vi "Set Source Debug Mode.vi"(5 "is Release?":bool=TRUE, 7 "Source Index":i32, 8 "error in (no error)":errorcluster, 11 "ProjectItem in":refnum<vi>) -> (0 "error out":errorcluster, 3 "ProjectItem out":refnum<vi>)   [LabVIEW 2019, in "Project Sync Tools.lvclass"]
uses:
  Project Sync Tools.lvclass
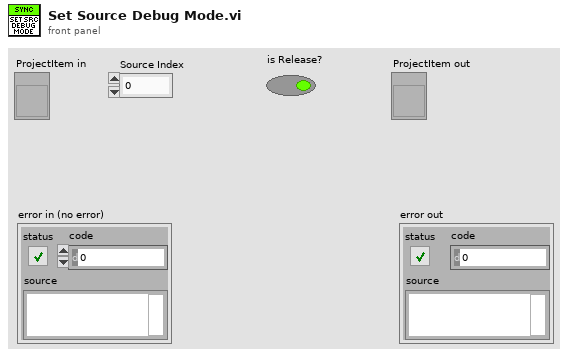
[diagram p1: front panel]
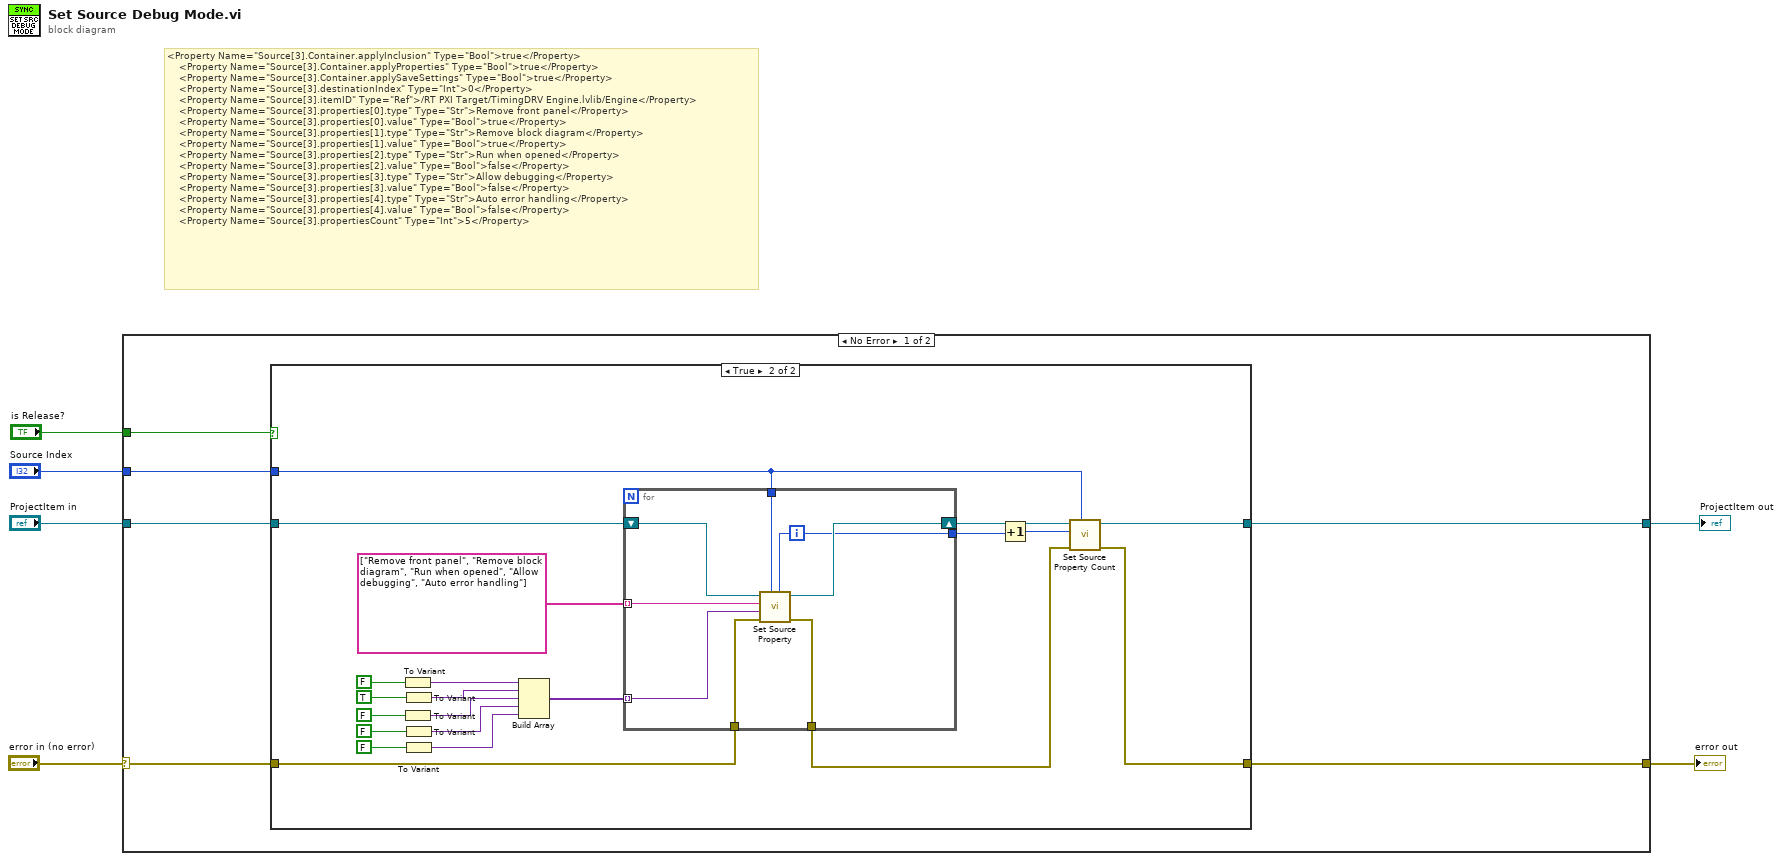
[diagram p0: block diagram]
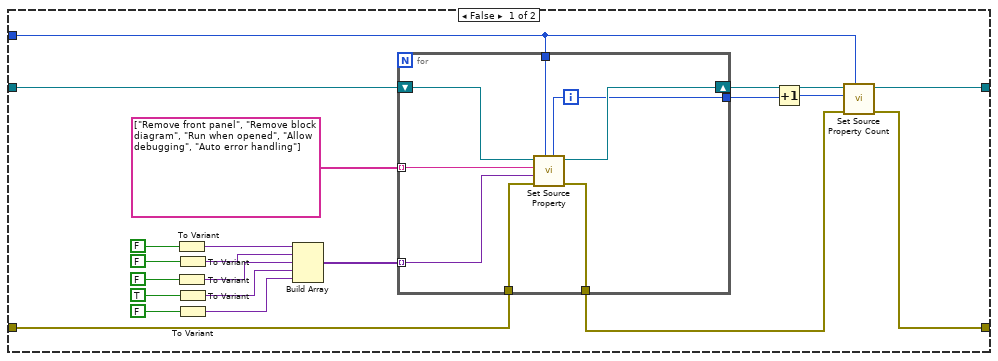
[diagram p2: hidden frame]
diagram:
  # "<Property Name=\"Source[3].Container.applyInclusion\" Type=\"Bool\">true</Property>\n\t\t\t\t<Property Name=\"Source[3].Container.applyProperties\" Type=\"Bool\">true</Property>\n\t\t\t\t<Property Name=\"Source[3].Container.applySaveSettings\" Type=\"Bool\">true</Property>\n\t\t\t\t<Property Name=\"Source[3].destinationIndex\" Type=\"Int\">0</Property>\n\t\t\t\t<Property Name=\"Source[3].itemID\" Type=\"Ref\">/RT PXI Target/TimingDRV Engine.lvlib/Engine</Property>\n\t\t\t\t<Property Name=\"Source[3].properties[0].type\" Type=\"Str\">Remove front panel</Property>\n\t\t\t\t<Property Name=\"Source[3].properties[0].value\" Type=\"Bool\">true</Property>\n\t\t\t\t<Property Name=\"Source[3].properties[1].type\" Type=\"Str\">Remove block diagram</Property>\n\t\t\t\t<Property Name=\"Source[3].properties[1].value\" Type=\"Bool\">true</Property>\n\t\t\t\t<Property Name=\"Source[3].properties[2].type\" Type=\"Str\">Run when opened</Property>\n\t\t\t\t<Property Name=\"Source[3].properties[2].value\" Type=\"Bool\">false</Property>\n\t\t\t\t<Property Name=\"Source[3].properties[3].type\" Type=\"Str\">Allow debugging</Property>\n\t\t\t\t<Property Name=\"Source[3].properties[3].value\" Type=\"Bool\">false</Property>\n\t\t\t\t<Property Name=\"Source[3].properties[4].type\" Type=\"Str\">Auto error handling</Property>\n\t\t\t\t<Property Name=\"Source[3].properties[4].value\" Type=\"Bool\">false</Property>\n\t\t\t\t<Property Name=\"Source[3].propertiesCount\" Type=\"Int\">5</Property>"
  n1 = case shown="No Error" "error in (no error)" {
    selector: "error in (no error)" -> [w11 w71]
    tunnel: "ProjectItem in" -> [w12 w72]
    tunnel: [w8 w71] -> w5
    tunnel: [w10 w72] -> w4
    tunnel: "Source Index" -> [w9 _]
    tunnel: "is Release?" -> [w7 _]
    frame No Error {
      n2 = case shown="True" w7 {
        tunnel: w12 -> [w17 w50]
        tunnel: w11 -> [w15 w49]
        tunnel: [w13 w47] -> w10
        tunnel: w9 -> [w16 w46]
        tunnel: [w14 w42] -> w8
        frame False {
          n3 = To Variant(anything=FALSE) -> (Variant=w27:variant)
          n4 = To Variant(anything=FALSE) -> (Variant=w25:variant)
          n5 = To Variant(anything=FALSE) -> (Variant=w26:variant)
          n6 = To Variant(anything=TRUE) -> (Variant=w24:variant)
          n7 = To Variant(anything=FALSE) -> (Variant=w23:variant)
          n8 = Build Array(w27, w26, w25, w24, w23) -> (w22:variant[])
          n9 = for {
            tunnel: string[] ["Remove front panel", "Remove block diagram", "Run when opened", "Allow debugging", "Auto error handling"] -> [w41] mode=indexing
            tunnel: w22 -> [w40] mode=indexing
            tunnel: w16 -> [w39]
            shift-right: [w37] -> w21
            shift-left: w17 -> [w38]
            tunnel: w15 -> [w36]
            tunnel: [w35] -> w18
            tunnel: [w34] -> w20
            i -> [w34]
            n10 = call "Set Source Property.vi"("Property Index"=w34, "Source Index"=w39, "error in (no error)"=w36, "Property Value"=w40, "Property Name"=w41, "BuildSpec in"=w38) -> ("error out"=w35:errorcluster, "BuildSpec out"=w37:refnum<vi>)  [unwired: 4 in]
          }
          n11 = Increment(x=w20) -> (x+1=w19:i32)
          n12 = call "Set Source Property Count.vi"("Source Index"=w16, "error in (no error)"=w18, "Properties Count"=w19, "BuildSpec in"=w21) -> ("error out"=w14:errorcluster, "BuildSpec out"=w13:refnum<vi>)  [unwired: 6 in]
        }
        frame True {
          n13 = To Variant(anything=FALSE) -> (Variant=w56:variant)
          n14 = To Variant(anything=FALSE) -> (Variant=w54:variant)
          n15 = To Variant(anything=TRUE) -> (Variant=w55:variant)
          n16 = To Variant(anything=FALSE) -> (Variant=w53:variant)
          n17 = To Variant(anything=FALSE) -> (Variant=w52:variant)
          n18 = Build Array(w56, w55, w54, w53, w52) -> (w51:variant[])
          n19 = for {
            tunnel: string[] ["Remove front panel", "Remove block diagram", "Run when opened", "Allow debugging", "Auto error handling"] -> [w70] mode=indexing
            tunnel: w51 -> [w69] mode=indexing
            tunnel: w46 -> [w68]
            shift-right: [w66] -> w48
            shift-left: w50 -> [w67]
            tunnel: w49 -> [w65]
            tunnel: [w64] -> w43
            tunnel: [w63] -> w45
            i -> [w63]
            n20 = call "Set Source Property.vi"("Property Index"=w63, "Source Index"=w68, "error in (no error)"=w65, "Property Value"=w69, "Property Name"=w70, "BuildSpec in"=w67) -> ("error out"=w64:errorcluster, "BuildSpec out"=w66:refnum<vi>)  [unwired: 4 in]
          }
          n21 = Increment(x=w45) -> (x+1=w44:i32)
          n22 = call "Set Source Property Count.vi"("Source Index"=w46, "error in (no error)"=w43, "Properties Count"=w44, "BuildSpec in"=w48) -> ("error out"=w42:errorcluster, "BuildSpec out"=w47:refnum<vi>)  [unwired: 6 in]
        }
      }
    }
    frame Error {
    }
  }
  "error out" <- w5
  "ProjectItem out" <- w4
